vi "Rotation Mount Global.vi"() -> ()   [LabVIEW 2012]
panel:
  out "Current Angle":dbl
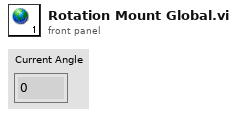
[diagram p1: front panel]
diagram:
